vi "Fatal.vi"(8 "Error In":errorcluster, 11 "Message":string) -> (0 "Error Out":errorcluster)   [LabVIEW 2025, in "LOGlib_LV2025.lvlib"]
doc: "Creates a logging statement from a message string with the FATAL level. The statement is created even if an error is passed to the Error In terminal. The level must be set to 1 or higher for this statement to be received by listeners. A logging statement is a comma-separated values (CSV) line containing an ISO 8601 timestamp, the level name (\"FATAL\"), the name of the origin VI, and the message."
uses:
  LOGlib_LV2025.lvlib
  Type Definitions/Tag.ctl
  Type Definitions/Statement.ctl
  Support/Action.ctl
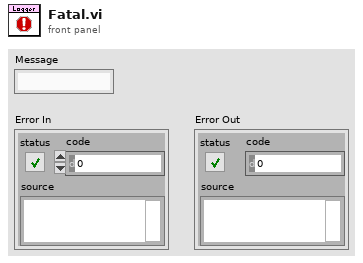
[diagram p1: front panel]
types:
  T1 = typedef "LOGlib_LV2025.lvlib/Tag.ctl" = enum16{"Fatal", "Error", "Warn", "Info", "Debug", "Trace"}
  T2 = typedef "LOGlib_LV2025.lvlib/Statement.ctl" = cluster{"Time Stamp":timestamp, "Tag":T1, "Source":string, "Message":string}
  T3 = typedef "LOGlib_LV2025.lvlib/Action.ctl" = enum16{"Initialize", "Register", "Log", "Unregister", "Set Level", "Shutdown"}
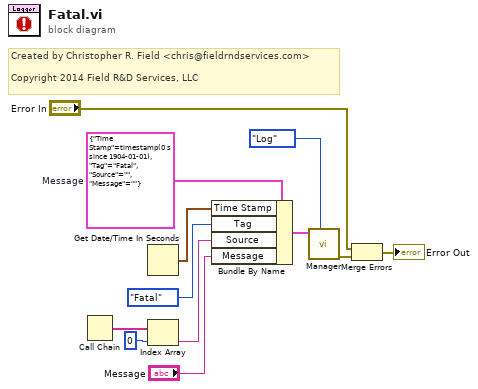
[diagram p0: block diagram]
diagram:
  w8 = T2 {"Time Stamp"=timestamp(0 s since 1904-01-01), "Tag"=enum."Fatal", "Source"="", "Message"=""}  # Message
  # "Created by Christopher R. Field <chris@fieldrndservices.com>\n\nCopyright 2014 Field R&D Services, LLC"
  n1 = Call Chain() -> (call chain=w10:string[])
  n2 = Get Date/Time In Seconds() -> (seconds since 1Jan1904=w7:timestamp)
  n3 = Index Array(array=w10, index=0) -> (element=w5:string)
  n4 = Bundle By Name(cluster=w8, "Time Stamp"=w7, "Tag"=Tag."Fatal" ("Level"), "Source"=w5, "Message"="Message") -> (w4:T2)
  n5 = call "Manager.vi"("Action"=Action."Log", "Value In"=w4) -> ("Error Out"=w3:errorcluster)  [unwired: 9 in]
  n6 = Merge Errors("Error In", w3) -> (→"Error Out":errorcluster)
